vi "Choose_Plug_In_to_Run.vi"(2 "setup":T1, 3 "Show Panel?":bool, 4 "Setup String In":string) -> (1 "Setup String Out":string)   [LabVIEW 2011]
uses:
  Anemometry Sub Vis/Controls/ok_button.ctl
  Anemometry Sub Vis/Controls/Setup.ctl
  Anemometry Sub Vis/Controls/Post_Process.ctl
  Anemometry Sub Vis/Globals/Meas_global.vi
  Anemometry Sub Vis/Globals/Dynamic_call_global.ph.vi
panel:
  out "Directories":path[](array[path])
  in  "Deselect Final":bool
  in  "Deselect per block":bool
  in  "Deselect Initial":bool
  in  "Override Post Process Plugins Setup":bool
  in  "OK Button":T2
  in  "Final Plug In":i32[](listbox)
  in  "Per Block Plug ins":i32[](listbox)
  in  "Initial Plug Ins":i32[](listbox)
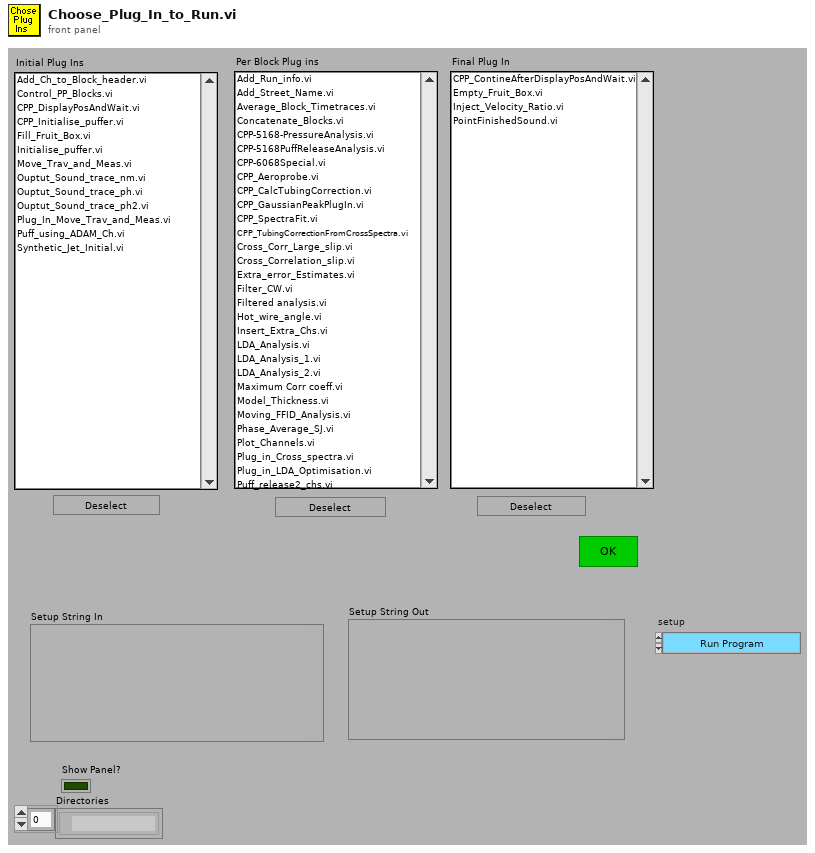
[diagram p1: front panel]
types:
  T1 = typedef "Setup.ctl" = enum16{"Run Program", "Show Setup", "Save Current Setup", "Setup Front Panel"}
  T2 = typedef "ok_button.ctl" = bool
  T3 = typedef "Post_Process.ctl" = enum16{"Take New Data", "Post Process Raw Data File"}
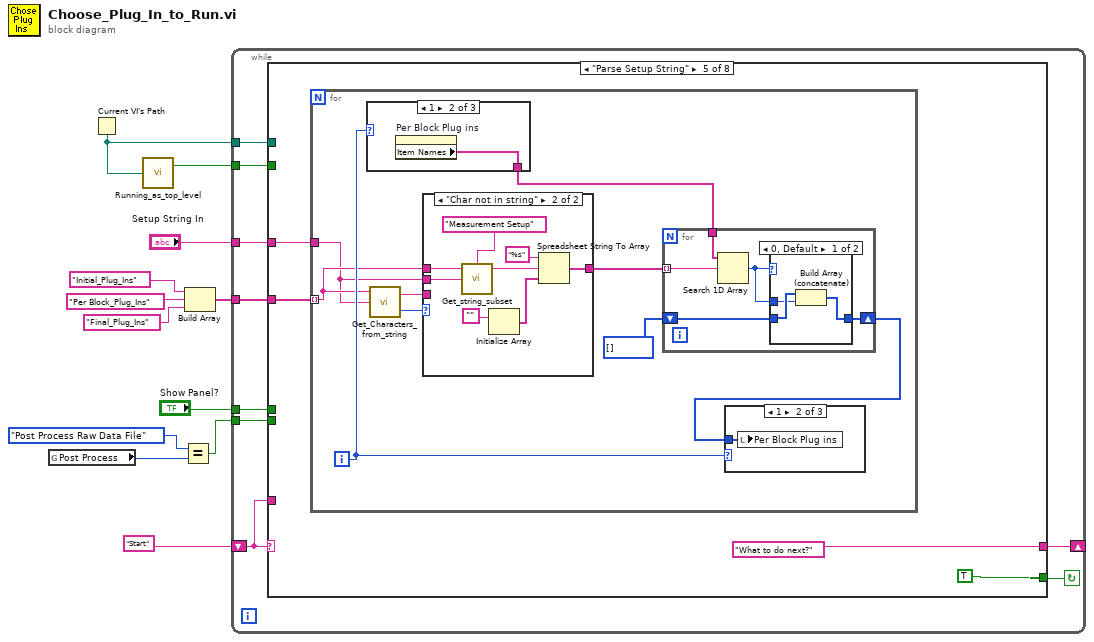
[diagram p0: block diagram]
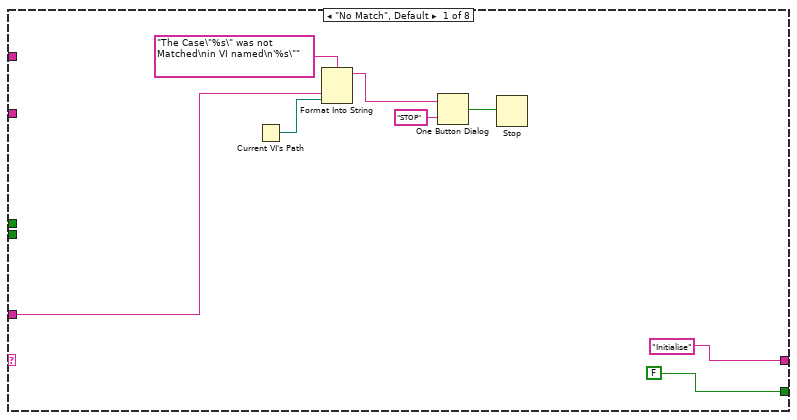
[diagram p2: hidden frame]
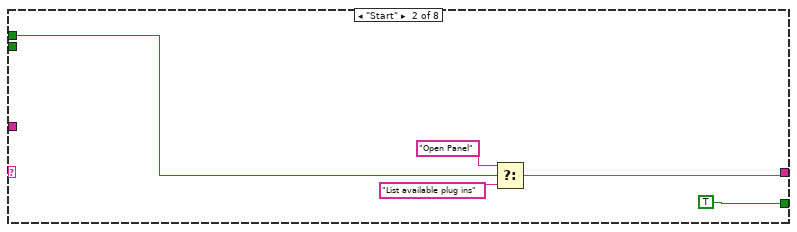
[diagram p3: hidden frame]
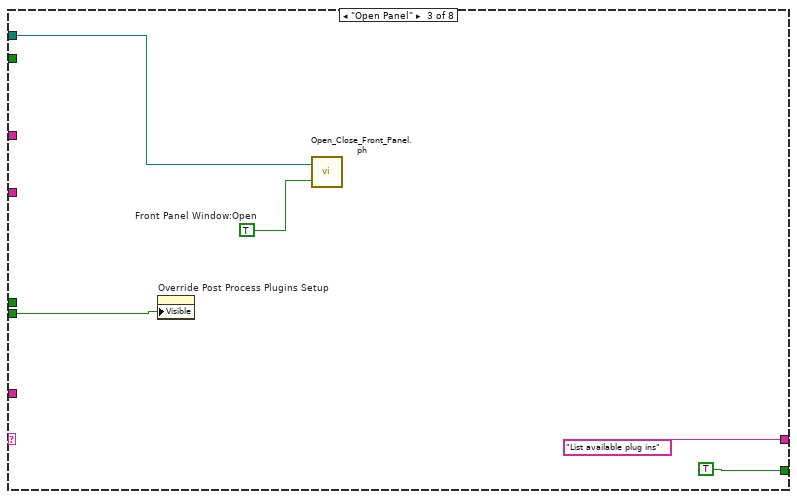
[diagram p4: hidden frame]
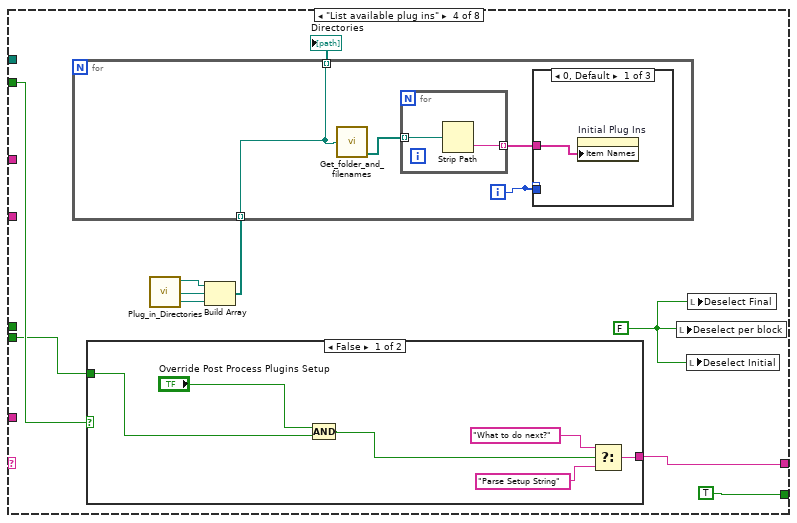
[diagram p5: hidden frame]
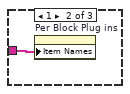
[diagram p6: hidden frame]
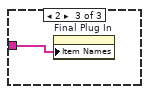
[diagram p7: hidden frame]
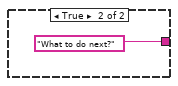
[diagram p8: hidden frame]
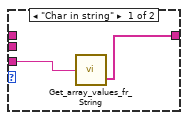
[diagram p9: hidden frame]
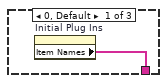
[diagram p11: hidden frame]
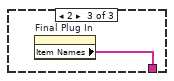
[diagram p12: hidden frame]
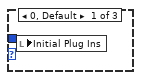
[diagram p13: hidden frame]
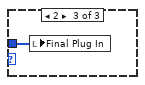
[diagram p14: hidden frame]
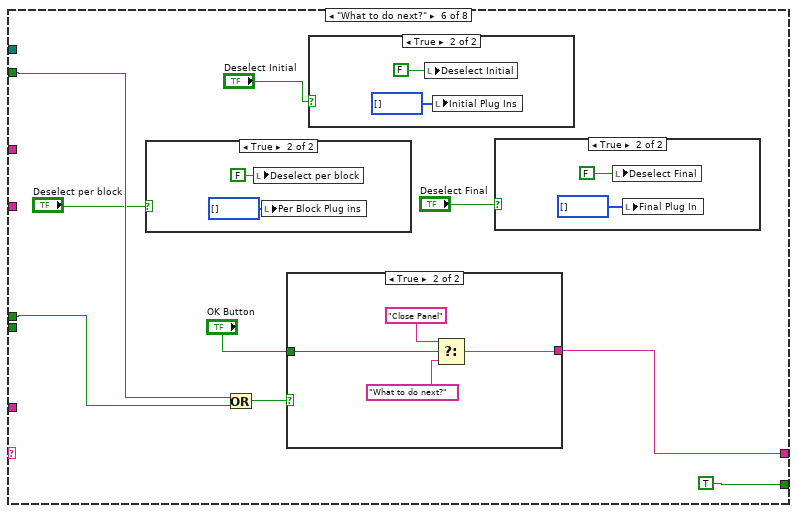
[diagram p15: hidden frame]
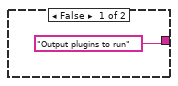
[diagram p19: hidden frame]
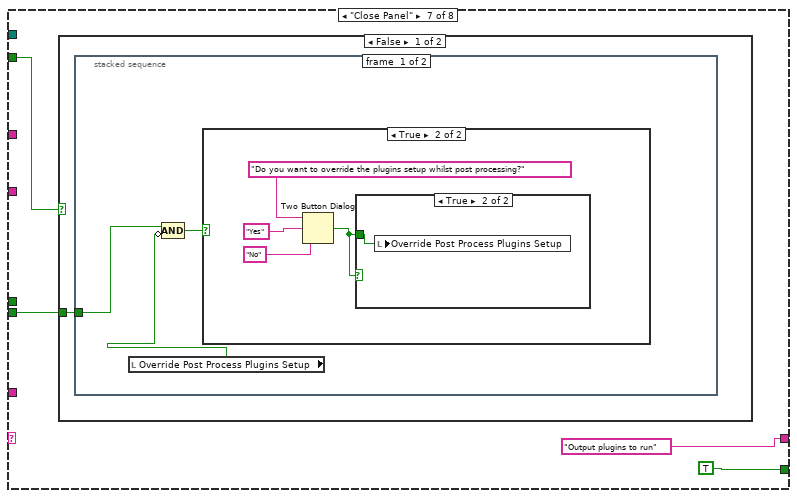
[diagram p20: hidden frame]
diagram:
  n1 = global read "Meas_global.vi" "Post Process"() -> (w2:T3)
  n2 = Current VI's Path() -> (path=w4:path)
  n3 = call "Running_as_top_level.vi"("Vi path name"=w4) -> ("Top Level"=w5:bool)  [unwired: 1 out]
  n4 = Equal?(x=Post_Process."Post Process Raw Data File" ("Post Process"), y=w2) -> (x = y?=w1:bool)
  n5 = Build Array("Initial_Plug_Ins", "Per Block_Plug_Ins", "Final_Plug_Ins") -> (w8:string[])
  n6 = while {
    shift-left: "Start" -> [w19]
    shift-right: [w20] -> _
    tunnel: w8 -> [w18]
    tunnel: "Show Panel?" -> [w17]
    tunnel: "Setup String In" -> [w16]
    tunnel: w5 -> [w15]
    tunnel: w4 -> [w14]
    tunnel: w1 -> [w13]
    stop <- w21 continue-if-true
    n7 = case shown="\"Parse Setup String\"" w19 {
      tunnel: [FALSE TRUE TRUE TRUE TRUE TRUE TRUE FALSE] -> w21
      tunnel: ["Initialise" w30 "List available plug ins" ("f") w48 "What to do next?" ("t") w110 "Output plugins to run" ("f") "End"] -> w20
      tunnel: w19 -> [w24 _ _ _ _ _ _ _]
      tunnel: w18 -> [_ _ _ _ w68 _ _ w153]
      tunnel: w17 -> [_ w32 _ _ _ w109 _ w150]
      tunnel: w16 -> [_ _ _ _ w67 _ _ w143]
      tunnel: w15 -> [_ _ _ w47 _ w108 w126 w149]
      tunnel: w14 -> [_ _ w36 _ _ _ _ _]
      tunnel: w13 -> [_ _ w35 w43 _ _ w124 w139]
      frame "No Match", Default {
        n8 = Current VI's Path() -> (path=w23:path)
        n9 = Format Into String(format string="The Case\"%s\" was not Matched\nin VI named\n'%s\"" ("Format String"), w24, w23) -> (resulting string=w27:string)  [unwired: 2 in, 1 out]
        n10 = One Button Dialog(message=w27, button name ("OK")="STOP") -> (true=w25:bool)
        n11 = Stop(stop? (T)=w25) -> ()
      }
      frame "Start" {
        n12 = Select(t="Open Panel", s=w32, f="List available plug ins") -> (s? t:f=w30:string)
      }
      frame "Open Panel" {
        w38 = TRUE  # Front Panel Window:Open
        n13 = property on="Override Post Process Plugins Setup" class="Bool (strict)"("Visible"=w35) -> ()  [unwired: 2 in, 2 out]
        n14 = call "Open_Close_Front_Panel.ph.vi"("Front Panel Window:Open"=w38, "VI path"=w36) -> ()  [unwired: 2 out]
      }
      frame "List available plug ins" {
        w46 = FALSE
        n15 = case shown="False" w47 {
          tunnel: [w60 "What to do next?"] -> w48
          tunnel: w43 -> [w59 _]
          frame False {
            n16 = Compound Arithmetic op=AND("Override Post Process Plugins Setup", w59) -> (w63:bool)
            n17 = Select(t="What to do next?", s=w63, f="Parse Setup String") -> (s? t:f=w60:string)
          }
          frame True {
          }
        }
        n18 = call "Plug_in_Directories.vi"() -> ("Final"=w40:path, "Per Block"=w41:path, "Initial"=w42:path)  [unwired: 1 out]
        n19 = Build Array(w42, w41, w40) -> (w45:path[])
        n20 = for {
          tunnel: w45 -> [w50] mode=indexing
          tunnel: [w50] -> w44 mode=indexing
          i -> [w52]
          n21 = call "Get_folder_and_filenames.vi"("file path (dialog if empty)"=w50) -> ("Files"=w53:path[])  [unwired: 1 out]
          n22 = for {
            tunnel: w53 -> [w58] mode=indexing
            tunnel: [w57] -> w51 mode=indexing
            n23 = Strip Path(path=w58) -> (name=w57:string)  [unwired: 1 out]
          }
          n24 = case shown="0, Default" w52 {
            tunnel: w52 -> [_ _ _]
            tunnel: w51 -> [w54 w55 w56]
            frame 0, Default {
              n25 = property on="Initial Plug Ins" class="LstBox (strict)"("Item Names"=w54) -> ()  [unwired: 2 in, 2 out]
            }
            frame 1 {
              n26 = property on="Per Block Plug ins" class="LstBox (strict)"("Item Names"=w55) -> ()  [unwired: 2 in, 2 out]
            }
            frame 2 {
              n27 = property on="Final Plug In" class="LstBox (strict)"("Item Names"=w56) -> ()  [unwired: 2 in, 2 out]
            }
          }
        }
        "Directories" <- w44
        n28 = local write "Deselect per block"(w46) -> ()
        n29 = local write "Deselect Initial"(w46) -> ()
        n30 = local write "Deselect Final"(w46) -> ()
      }
      frame "Parse Setup String" {
        n31 = for {
          tunnel: w68 -> [w74] mode=indexing
          tunnel: w67 -> [w73]
          i -> [w76]
          n32 = case shown="1" w76 {
            tunnel: [w98 w99 w100] -> w75
            frame 0, Default {
              n33 = property on="Initial Plug Ins" class="LstBox (strict)"() -> ("Item Names"=w98:string[])  [unwired: 2 in, 2 out]
            }
            frame 1 {
              n34 = property on="Per Block Plug ins" class="LstBox (strict)"() -> ("Item Names"=w99:string[])  [unwired: 2 in, 2 out]
            }
            frame 2 {
              n35 = property on="Final Plug In" class="LstBox (strict)"() -> ("Item Names"=w100:string[])  [unwired: 2 in, 2 out]
            }
          }
          n36 = call "Get_Characters_from_string.vi"("Input string"=w73, "Variable name"=w74) -> ("Status"=w71:enum16{"Char in string", "Char not in string"}, "Value"=w70:string)  [unwired: 1 in]
          n37 = case shown="\"Char not in string\"" w71 {
            tunnel: w74 -> [_ w88]
            tunnel: w73 -> [_ w87]
            tunnel: [w79 w83] -> w72
            tunnel: w70 -> [w80 _]
            frame "Char in string" {
              n38 = call "Get_array_values_fr_String.vi"("String Value"=w80) -> ("String array"=w79:string[])  [unwired: 1 out]
            }
            frame "Char not in string" {
              n39 = call "Get_string_subset.vi"("String Name"="Measurement Setup", "String to split"=w87, "File Label"=w88) -> ("Output string"=w82:string)  [unwired: 1 in, 1 out]
              n40 = Initialize Array("") -> (w86:string[])  [unwired: 1 out]
              n41 = Spreadsheet String To Array(format string="%s", spreadsheet string=w82, array type (2D Dbl)=w86) -> (array=w83:string[])  [unwired: 1 out]
            }
          }
          n42 = for {
            tunnel: w75 -> [w93]
            tunnel: w72 -> [w92] mode=indexing
            shift-right: [w91] -> w77
            shift-left: i32[] [] -> [w90]
            n43 = Search 1D Array(1D array=w93, element=w92) -> (index of element=w89:i32)  [unwired: 1 out]
            n44 = case shown="0, Default" w89 {
              tunnel: [w94 w97] -> w91
              tunnel: w90 -> [w96 w97]
              tunnel: w89 -> [w95 _]
              frame 0, Default {
                n45 = Build Array (concatenate)(w96, w95) -> (w94:i32[])
              }
              frame -1 {
              }
            }
          }
          n46 = case shown="1" w76 {
            tunnel: w77 -> [w101 w102 w103]
            frame 0, Default {
              n47 = local write "Initial Plug Ins"(w101) -> ()
            }
            frame 1 {
              n48 = local write "Per Block Plug ins"(w102) -> ()
            }
            frame 2 {
              n49 = local write "Final Plug In"(w103) -> ()
            }
          }
        }
      }
      frame "What to do next?" {
        n50 = case shown="True" "Deselect per block" {
          frame False {
          }
          frame True {
            n51 = local write "Deselect per block"(FALSE ("Deselect Initial")) -> ()
            n52 = local write "Per Block Plug ins"(i32[] [] ("Initial Plug Ins")) -> ()
          }
        }
        n53 = Or(x=w108, y=w109) -> (x .or. y?=w107:bool)
        n54 = case shown="True" w107 {
          tunnel: "OK Button" -> [_ w123]
          tunnel: ["Output plugins to run" w120] -> w110
          frame False {
          }
          frame True {
            n55 = Select(t="Close Panel", s=w123, f="What to do next?") -> (s? t:f=w120:string)
          }
        }
        n56 = case shown="True" "Deselect Initial" {
          frame False {
          }
          frame True {
            n57 = local write "Deselect Initial"(FALSE ("Deselect Initial")) -> ()
            n58 = local write "Initial Plug Ins"(i32[] [] ("Initial Plug Ins")) -> ()
          }
        }
        n59 = case shown="True" "Deselect Final" {
          frame False {
          }
          frame True {
            n60 = local write "Deselect Final"(FALSE ("Deselect Initial")) -> ()
            n61 = local write "Final Plug In"(i32[] [] ("Initial Plug Ins")) -> ()
          }
        }
      }
      frame "Close Panel" {
        n62 = case shown="False" w126 {
          tunnel: w124 -> [w128 _]
          frame False {
            n63 = stacked-sequence {
              tunnel: w128 -> [w129 _]
              frame #0 {
                n64 = local read "Override Post Process Plugins Setup"() -> (w131:bool)
                n65 = Compound Arithmetic op=AND(w129, invert w131) -> (w130:bool)
                n66 = case shown="True" w130 {
                  frame False {
                  }
                  frame True {
                    n67 = Two Button Dialog(message="Do you want to override the plugins setup whilst post processing?", 1:"No" ("F button name (\"Cancel\")"), 2:"Yes" ("T button name (\"OK\")")) -> (T button?=w134:bool)
                    n68 = case shown="True" w134 {
                      tunnel: w134 -> [_ w136]
                      frame False {
                      }
                      frame True {
                        n69 = local write "Override Post Process Plugins Setup"(w136) -> ()
                      }
                    }
                  }
                }
              }
              frame #1 {
                w138 = FALSE  # Front Panel Window:Open
                n70 = Current VI's Path() -> (path=w137:path)
                n71 = call "Open_Close_Front_Panel.ph.vi"("Front Panel Window:Open"=w138, "VI path"=w137) -> ()  [unwired: 2 out]
              }
            }
          }
          frame True {
          }
        }
      }
      frame "Output plugins to run" {
        n72 = Or(x=w149, y=w150) -> (x .or. y?=w148:bool)
        n73 = Select(t=w143, s=w150, f="") -> (s? t:f=w142:string)
        n74 = local read "Override Post Process Plugins Setup"() -> (w141:bool)
        n75 = local read "Directories"() -> (w154:path[])
        n76 = for {
          shift-right: [w159] -> w145
          shift-left: w142 -> [w157]
          tunnel: w154 -> [w165] mode=indexing
          tunnel: w153 -> [w158] mode=indexing
          tunnel: "setup" -> [w164]
          tunnel: w148 -> [w161]
          i -> [w166]
          n77 = case shown="2" w166 {
            tunnel: ["Initial Plug Ins" "Per Block Plug ins" "Final Plug In"] -> w167
            tunnel: [w173 w175 w177] -> w160
            frame 0, Default {
              n78 = property on="Initial Plug Ins" class="LstBox (strict)"() -> ("Item Names"=w173:string[])  [unwired: 2 in, 2 out]
            }
            frame 1 {
              n79 = property on="Per Block Plug ins" class="LstBox (strict)"() -> ("Item Names"=w175:string[])  [unwired: 2 in, 2 out]
            }
            frame 2 {
              n80 = property on="Final Plug In" class="LstBox (strict)"() -> ("Item Names"=w177:string[])  [unwired: 2 in, 2 out]
            }
          }
          n81 = for {
            tunnel: w167 -> [w187] mode=indexing
            tunnel: w165 -> [w186]
            tunnel: [w180] -> w162 mode=indexing
            tunnel: w161 -> [w185]
            tunnel: w160 -> [w183]
            shift-right: [w181] -> w155
            shift-left: "" -> [w182]
            n82 = Index Array(array=w183, index=w187) -> (element=w180:string)
            n83 = Build Path(base path=w186, name or relative path=w180) -> (appended path=w184:path)
            n84 = case shown="True" w185 {
              tunnel: w184 -> [_ w196]
              frame False {
              }
              frame True {
                n85 = Open VI Reference(vi path=w196) -> (vi reference=w193:refnum<vi>, error out=w192:errorcluster)  [unwired: 1 in, 4 out]
                n86 = invoke class="VI" method="FP.Old Open"(reference=w193, error in=w192) -> (reference out=w191:refnum<vi>, error out=w190:errorcluster)  [unwired: 3 in, 3 out]
                n87 = invoke class="VI" method="Run VI"(reference=w191, error in=w190, "Wait until done"=FALSE, "Auto Dispose Ref"=TRUE) -> (reference out=w189:refnum<vi>, error out=w188:errorcluster)  [unwired: 1 in, 3 out]
                n88 = Close Reference(reference=w189, error in (no error)=w188) -> ()  [unwired: 1 out]
              }
            }
            n89 = Concatenate Strings(w182, w180, ";" ("string")) -> (w181:string)
          }
          n90 = case shown="\"Show Setup\", Default" w164 {
            tunnel: [w168 string[] []] -> w163
            tunnel: w162 -> [w168 _]
            frame "Run Program" {
            }
            frame "Show Setup", Default {
            }
          }
          n91 = case shown="2" w166 {
            tunnel: w163 -> [w170 w171 w172]
            frame 0, Default {
              n92 = global write "Dynamic_call_global.ph.vi" "Initial Plug Ins"(w170) -> ()
            }
            frame 1 {
              n93 = global write "Dynamic_call_global.ph.vi" "Per Block Plug Ins"(w171) -> ()
            }
            frame 2 {
              n94 = global write "Dynamic_call_global.ph.vi" "Final Plug Ins"(w172) -> ()
            }
          }
          n95 = call "Replace_data_in_setup_string.vi"("New data string"=w155, "Input string"=w157, "Variable name"=w158) -> ("Appended string"=w159:string)
        }
        n96 = Compound Arithmetic op=OR(w141, invert w139) -> (w140:bool)
        n97 = Select(t=w145, s=w140, f=w142) -> (s? t:f=→"Setup String Out":string)
      }
    }
  }
